vi "validate_queue.vi"(1 "Queue":string[][](table)=[["Formula", "Start", "Finish", "Points", "Time"], ["t", "3", "5", "100", "600"], ["", "", "", "", ""]], 2 "Max Sweep Rates":dbl[][](array[numeric])) -> (0 "Valid?":bool)   [LabVIEW 2016]
uses:
  <vilib>/gmath/NI_Gmath.lvlib
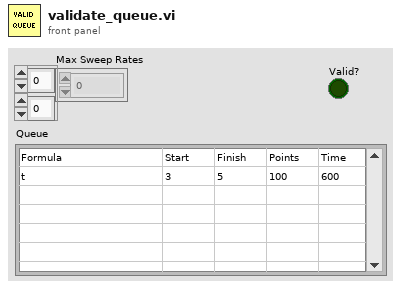
[diagram p1: front panel]
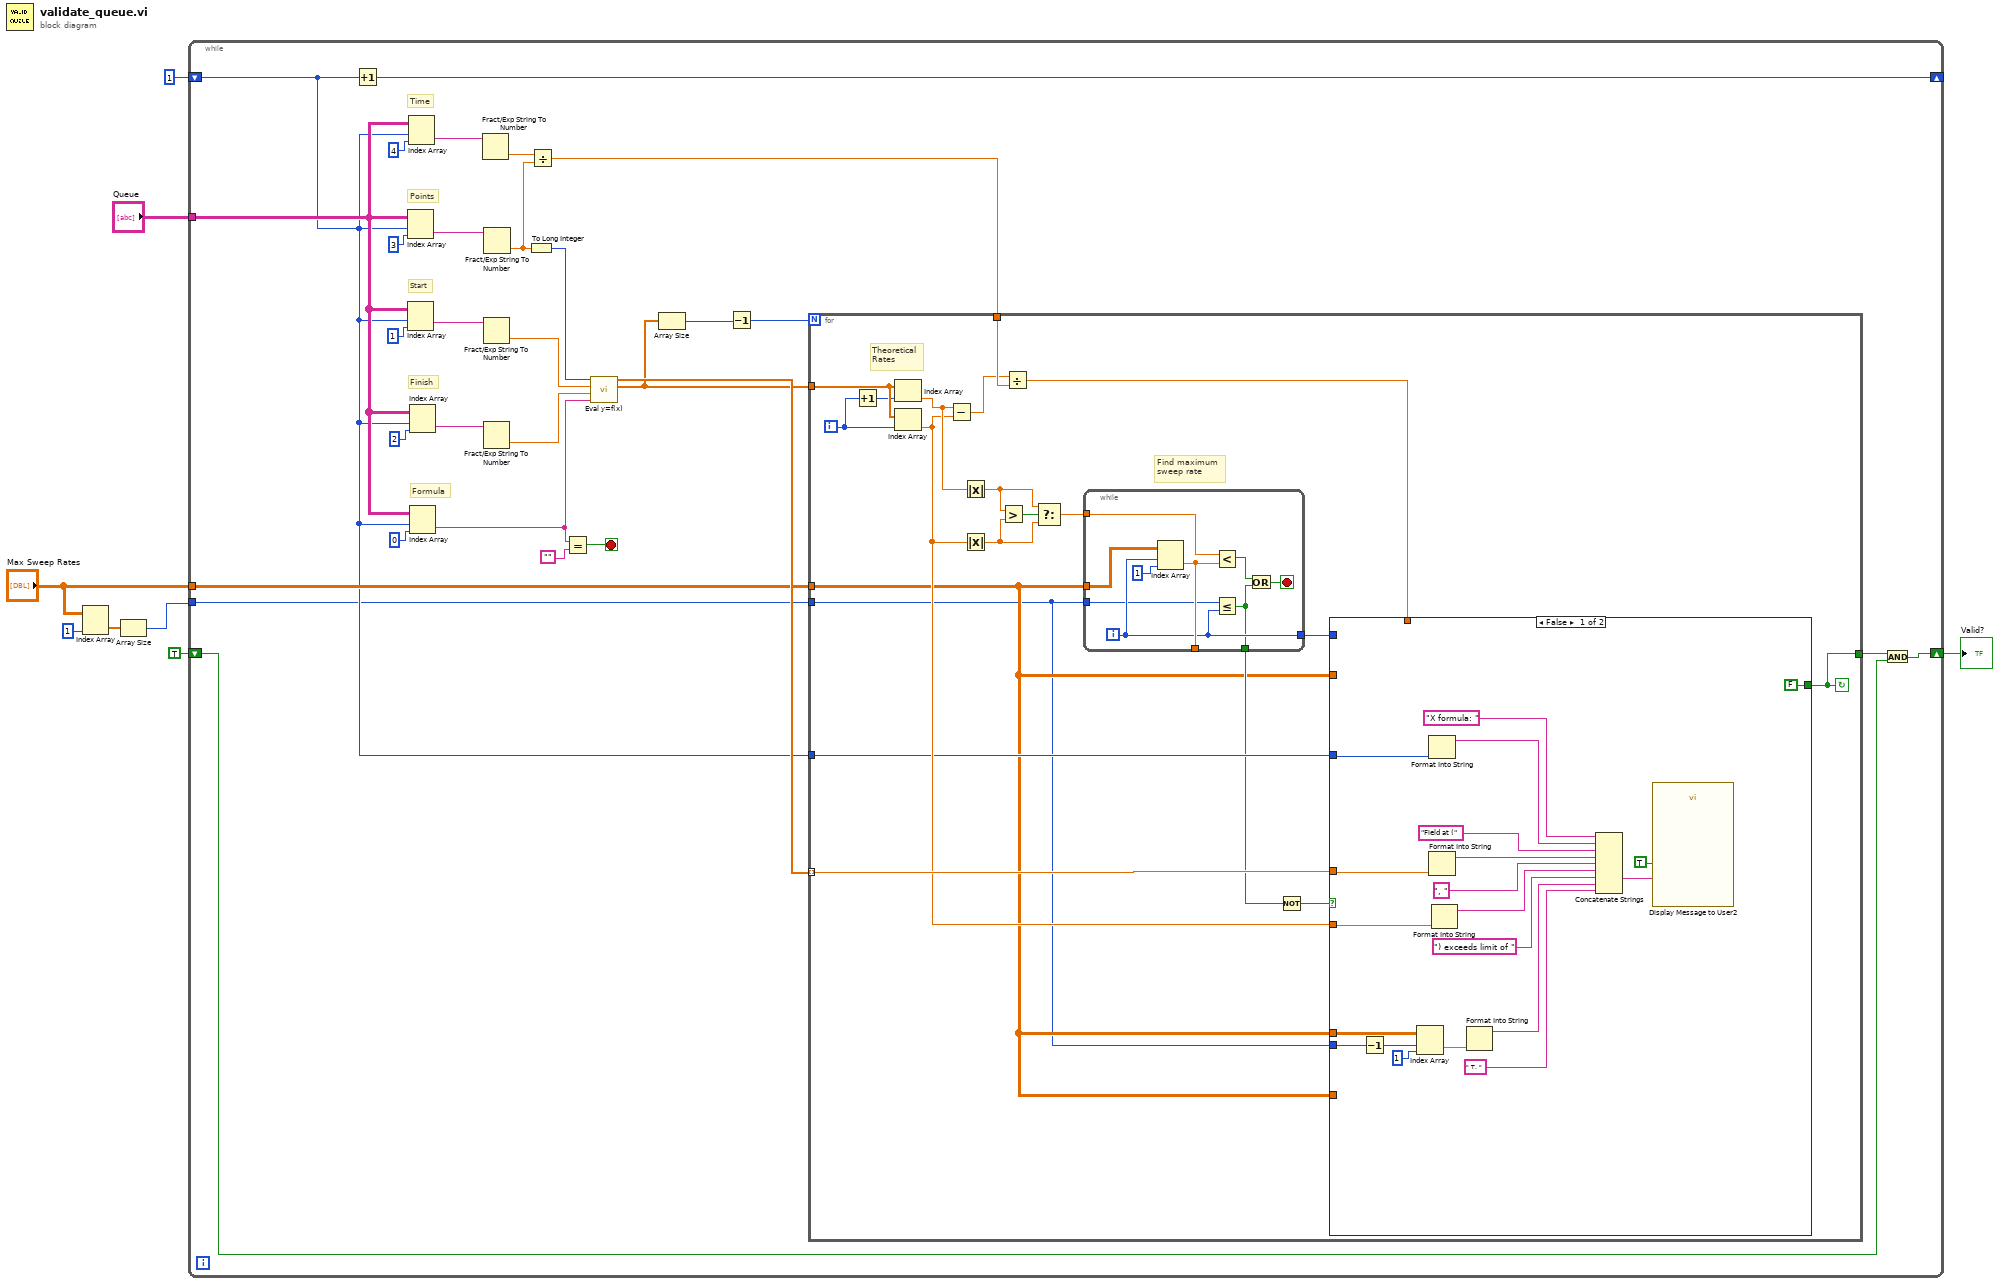
[diagram p0: block diagram]
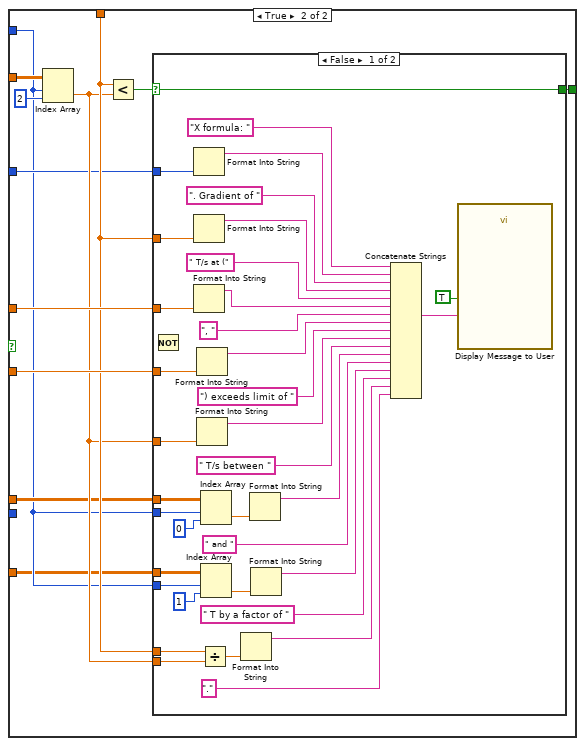
[diagram p2: hidden frame]
diagram:
  n1 = Index Array(array="Max Sweep Rates", index (col)=1 ("index (row)")) -> (element=w2:dbl[])  [unwired: 1 in]
  n2 = Array Size(array=w2) -> (size(s)=w1:i32)
  n3 = while {
    tunnel: "Queue" -> [w22]
    tunnel: "Max Sweep Rates" -> [w19]
    shift-right: [w14] -> _
    shift-left: 1 ("disabled index (col)") -> [w15]
    shift-right: [w12] -> w6
    shift-left: TRUE -> [w10]
    tunnel: w1 -> [w9]
    stop <- w13 stop-if-true
    # "Time"
    # "Points"
    # "Formula"
    # "Finish"
    # "Start"
    n4 = Increment(x=w15) -> (x+1=w14:i32)
    n5 = Index Array(array=w22, index (row)=w15, index (col)=3 ("disabled index (col)")) -> (element=w32:string)
    n6 = Index Array(array=w22, index (row)=w15, index (col)=1) -> (element=w35:string)
    n7 = Index Array(array=w22, index (row)=w15, index (col)=4) -> (element=w27:string)
    n8 = Index Array(array=w22, index (row)=w15, index (col)=2) -> (element=w34:string)
    n9 = Index Array(array=w22, index (row)=w15, index (col)=0) -> (element=w17:string)
    n10 = Fract/Exp String To Number(string=w27) -> (number=w26:dbl)  [unwired: 3 in, 1 out]
    n11 = Fract/Exp String To Number(string=w35) -> (number=w31:dbl)  [unwired: 3 in, 1 out]
    n12 = Fract/Exp String To Number(string=w34) -> (number=w30:dbl)  [unwired: 3 in, 1 out]
    n13 = Fract/Exp String To Number(string=w32) -> (number=w25:dbl)  [unwired: 3 in, 1 out]
    n14 = To Long Integer(number=w25) -> (32bit integer=w18:i32)
    n15 = Divide(x=w26, y=w25) -> (x/y=w20:dbl)
    n16 = Equal?(x=w17, y="") -> (x = y?=w13:bool)
    n17 = call <vilib>:"Eval y=f(x).vi"("formula"=w17, "end"=w30, "start"=w31, "number of points"=w18) -> ("Y Values"=w21:dbl[], "X Values"=w24:dbl[])  [unwired: 2 out]
    n18 = Array Size(array=w21) -> (size(s)=w23:i32)
    n19 = Decrement(x=w23) -> (x-1=w29:i32)
    n20 = for {
      N: w29 -> [_]
      tunnel: w21 -> [w58]
      tunnel: w20 -> [w55]
      tunnel: w24 -> [w48] mode=indexing
      tunnel: w19 -> [w40]
      tunnel: w15 -> [w44]
      tunnel: [w43] -> w11
      tunnel: w9 -> [w39]
      i -> [w56]
      stop <- w43 continue-if-true
      # "Find maximum\nsweep rate"
      # "Theoretical\nRates"
      n21 = Increment(x=w56) -> (x+1=w57:i32)
      n22 = Index Array(array=w58, index=w57) -> (element=w49:dbl)
      n23 = Index Array(array=w58, index=w56) -> (element=w47:dbl)
      n24 = Subtract(x=w49, y=w47) -> (x-y=w54:dbl)
      n25 = Absolute Value(x=w49) -> (abs(x)=w51:dbl)
      n26 = Absolute Value(x=w47) -> (abs(x)=w52:dbl)
      n27 = Greater?(x=w51, y=w52) -> (0:w53:bool)
      n28 = Divide(x=w54, y=w55) -> (x/y=w45:dbl)
      n29 = Select(t=w51, s=w53, f=w52) -> (s? t:f=w50:dbl)
      n30 = while {
        tunnel: w40 -> [w133]
        tunnel: w50 -> [w135]
        tunnel: [w132] -> w46
        tunnel: [w134] -> _
        tunnel: w39 -> [w129]
        tunnel: [w128] -> w41
        i -> [w132]
        stop <- w130 stop-if-true
        n31 = Index Array(array=w133, index (row)=w132, index (col)=1 ("disabled index (col)")) -> (element=w134:dbl)
        n32 = Less?(x=w135, y=w134) -> (x < y?=w131:bool)
        n33 = Less Or Equal?(x=w129, y=w132) -> (x <= y?=w128:bool)
        n34 = Or(x=w131, y=w128) -> (x .or. y?=w130:bool)
      }
      n35 = Not(x=w41) -> (.not. x?=w42:bool)
      n36 = case shown="False" w42 {
        tunnel: w48 -> [w65 w88]
        tunnel: w47 -> [w64 w87]
        tunnel: w46 -> [_ w80]
        tunnel: w45 -> [_ w86]
        tunnel: w40 -> [_ w84]
        tunnel: w44 -> [w66 w83]
        tunnel: [FALSE w82] -> w43
        tunnel: w40 -> [w61 w81]
        tunnel: w40 -> [_ w79]
        tunnel: w39 -> [w59 _]
        frame False {
          n37 = Decrement(x=w59) -> (x-1=w60:i32)
          n38 = Index Array(array=w61, index (row)=w60, index (col)=1 ("disabled index (col)")) -> (element=w62:dbl)
          n39 = Format Into String(w66) -> (resulting string=w68:string)  [unwired: 3 in, 1 out]
          n40 = Format Into String(w65) -> (resulting string=w74:string)  [unwired: 3 in, 1 out]
          n41 = Format Into String(w64) -> (resulting string=w72:string)  [unwired: 3 in, 1 out]
          n42 = Format Into String(w62) -> (resulting string=w70:string)  [unwired: 3 in, 1 out]
          n43 = Concatenate Strings("X formula: " ("Message"), w68, "Field at (" ("Message"), w74, ", " ("Message"), w72, ") exceeds limit of " ("Message"), w70, " T. " ("Message")) -> (w76:string)
          n44 = call "Display Message to User2"("Enable"=TRUE, "Message"=w76) -> ()  [unwired: 8 in, 2 out]
        }
        frame True {
          n45 = Index Array(array=w84, index (row)=w80, index (col)=2 ("disabled index (col)")) -> (element=w85:dbl)
          n46 = Less?(x=w86, y=w85) -> (x < y?=w89:bool)
          n47 = case shown="False" w89 {
            selector: w89 -> [w126 w127]
            tunnel: [w126 w127] -> w82
            tunnel: w86 -> [w122 _]
            tunnel: w88 -> [w119 _]
            tunnel: w87 -> [w116 _]
            tunnel: w85 -> [w113 _]
            tunnel: w80 -> [w109 _]
            tunnel: w81 -> [w108 _]
            tunnel: w86 -> [w102 _]
            tunnel: w85 -> [w101 _]
            tunnel: w83 -> [w95 _]
            tunnel: w80 -> [w94 _]
            tunnel: w79 -> [w93 _]
            frame False {
              n48 = Not() -> ()  [unwired: 1 in, 1 out]
              n49 = Format Into String(w95) -> (resulting string=w97:string)  [unwired: 3 in, 1 out]
              n50 = Format Into String(w122) -> (resulting string=w121:string)  [unwired: 3 in, 1 out]
              n51 = Format Into String(w119) -> (resulting string=w118:string)  [unwired: 3 in, 1 out]
              n52 = Format Into String(w116) -> (resulting string=w115:string)  [unwired: 3 in, 1 out]
              n53 = Format Into String(w113) -> (resulting string=w112:string)  [unwired: 3 in, 1 out]
              n54 = Divide(x=w102, y=w101) -> (x/y=w100:dbl)
              n55 = Index Array(array=w108, index (row)=w109, index (col)=0 ("disabled index (col)")) -> (element=w107:dbl)
              n56 = Index Array(array=w93, index (row)=w94, index (col)=1 ("disabled index (col)")) -> (element=w91:dbl)
              n57 = Format Into String(w100) -> (resulting string=w99:string)  [unwired: 3 in, 1 out]
              n58 = Format Into String(w107) -> (resulting string=w106:string)  [unwired: 3 in, 1 out]
              n59 = Format Into String(w91) -> (resulting string=w104:string)  [unwired: 3 in, 1 out]
              n60 = Concatenate Strings("X formula: " ("Message"), w97, ". Gradient of " ("Message"), w121, " T/s at (" ("Message"), w118, ", " ("Message"), w115, ") exceeds limit of " ("Message"), w112, " T/s between " ("Message"), w106, " and " ("Message"), w104, " T by a factor of " ("Message"), w99, "." ("Message")) -> (w124:string)
              n61 = call "Display Message to User"("Enable"=TRUE, "Message"=w124) -> ()  [unwired: 8 in, 2 out]
            }
            frame True {
            }
          }
        }
      }
    }
    n62 = And(x=w11, y=w10) -> (x .and. y?=w12:bool)
  }
  "Valid?" <- w6
